vi "OSICS_Wait_for_OPC_GPIB.vi"(8 "error in":errorcluster, 10 "Timeout (s)":sgl=60.0, 11 "VISA IN":refnum<visa-resource-name>) -> (0 "error out":errorcluster, 2 "ERR":i32, 3 "VISA OUT":refnum<visa-resource-name>)   [LabVIEW 2014, in "OSICS_LIB.lvlib"]
doc: "This Vi checks the status byte register until the OPC byte is asserted or timeout is reached, what ever comes first. It then generates an Error Code ERR if any error were detected in the STB.\nGPIB only."
uses:
  OSICS_LIB.lvlib
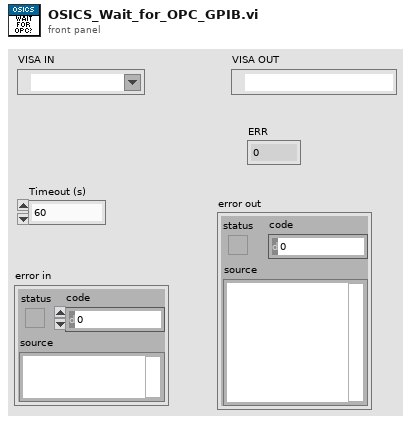
[diagram p1: front panel]
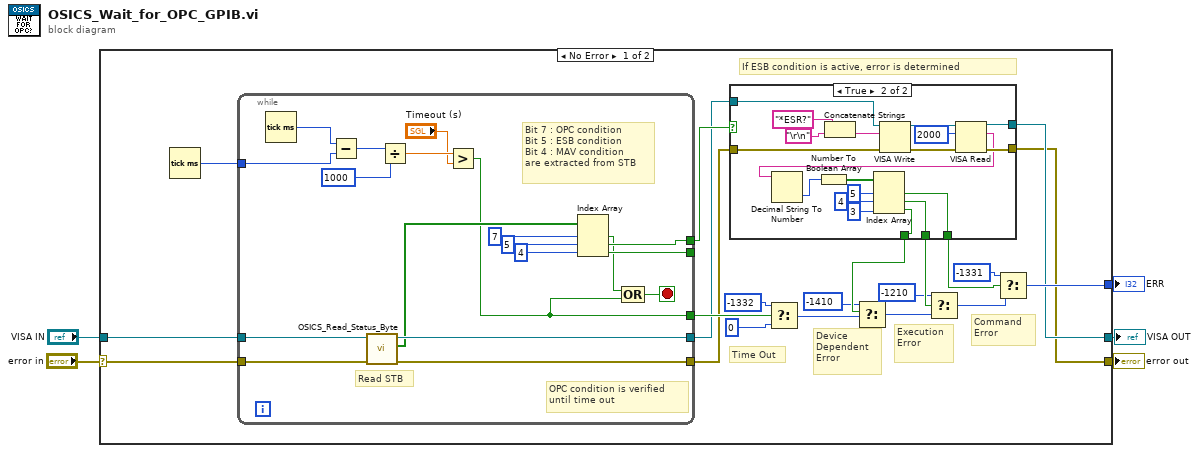
[diagram p0: block diagram]
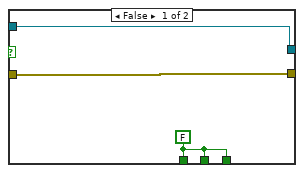
[diagram p2: hidden frame]
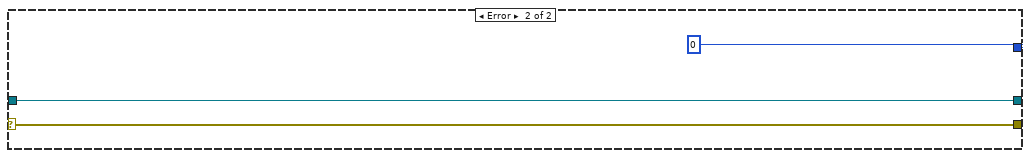
[diagram p3: hidden frame]
diagram:
  n1 = case shown="No Error" "error in" {
    selector: "error in" -> [w20 w70]
    tunnel: "VISA IN" -> [w26 w69]
    tunnel: [w14 w70] -> w4
    tunnel: [w15 w69] -> w3
    tunnel: [w19 0 ("f")] -> w1
    frame No Error {
      # "If ESB condition is active, error is determined"
      # "Device\nDependent\nError"
      # "Command\nError"
      # "Execution Error"
      # "Time Out"
      n2 = Tick Count (ms)() -> (millisecond timer value=w6:u32)
      n3 = while {
        tunnel: w26 -> [w63]
        tunnel: w20 -> [w56]
        tunnel: [w66] -> w16
        tunnel: [w67] -> w17
        tunnel: [w49] -> w22
        tunnel: [w65] -> w18
        tunnel: [w64] -> _
        tunnel: w6 -> [w54]
        stop <- w61 stop-if-true
        # "Read STB"
        # "OPC condition is verified\nuntil time out"
        # "Bit 7 : OPC condition\nBit 5 : ESB condition\nBit 4 : MAV condition\nare extracted from STB"
        n4 = Tick Count (ms)() -> (millisecond timer value=w55:u32)
        n5 = Subtract(x=w55, y=w54) -> (x-y=w53:u32)
        n6 = call "OSICS_Read_Status_Byte.vi"("error in"=w56, "VISA IN"=w63) -> ("error out"=w66:errorcluster, "SBR"=w62:bool[], "VISA OUT"=w67:refnum<visa-resource-name>)  [unwired: 7 in]
        n7 = Divide(x=w53, y=u32 1000) -> (x/y=w51:dbl)
        n8 = Greater?(x=w51, y="Timeout (s)") -> (0:w49:bool)
        n9 = Index Array(array=w62, index #1=7 ("index"), index #2=5 ("index"), index #3=4 ("index")) -> (element #1=w57:bool, element #2=w65:bool, element #3=w64:bool)
        n10 = Compound Arithmetic op=OR(w57, w49) -> (w61:bool)
      }
      n11 = case shown="True" w18 {
        tunnel: w16 -> [w29 w42]
        tunnel: w17 -> [w28 w41]
        tunnel: [w28 w40] -> w15
        tunnel: [w29 w39] -> w14
        tunnel: [w27 w33] -> w13
        tunnel: [w27 w32] -> w12
        tunnel: [w27 w31] -> w8
        frame False {
          w27 = FALSE
        }
        frame True {
          n12 = Concatenate Strings("*ESR?" ("string"), "\r\n") -> (w47:string)
          n13 = VISA Write(VISA resource name=w41, write buffer=w47, error in (no error)=w42) -> (VISA resource name out=w44:refnum<visa-resource-name>, error out=w45:errorcluster)  [unwired: 1 out]
          n14 = VISA Read(VISA resource name=w44, byte count=u32 2000, error in (no error)=w45) -> (VISA resource name out=w40:refnum<visa-resource-name>, read buffer=w38:string, error out=w39:errorcluster)  [unwired: 1 out]
          n15 = Decimal String To Number(string=w38) -> (number=w30:i32)  [unwired: 2 in, 1 out]
          n16 = Number To Boolean Array(number=w30) -> (Boolean array=w37:bool[])
          n17 = Index Array(array=w37, index #1=5 ("index"), index #2=4 ("index"), index #3=3 ("index")) -> (element #1=w33:bool, element #2=w32:bool, element #3=w31:bool)
        }
      }
      n18 = Select(t=-1332, s=w22, f=0) -> (s? t:f=w10:i32)
      n19 = Select(t=-1410, s=w8, f=w10) -> (s? t:f=w9:i32)
      n20 = Select(t=-1210, s=w12, f=w9) -> (s? t:f=w25:i32)
      n21 = Select(t=-1331, s=w13, f=w25) -> (s? t:f=w19:i32)
    }
    frame Error {
    }
  }
  "error out" <- w4
  "VISA OUT" <- w3
  "ERR" <- w1
